vi "LVCAM Propagate Error.vi"(10 "error in":errorcluster, 11 "LVCAM Propagate Error in":refnum<class "LVCAM Propagate Error.lvclass">) -> (0 "error out":errorcluster, 3 "LVCAM Propagate Error out":refnum<class "LVCAM Propagate Error.lvclass">)   [LabVIEW 2021, in "LVCAM.lvlib" / "LVCAM Propagate Error.lvclass"]
uses:
  LVCAM Propagate Error.lvclass
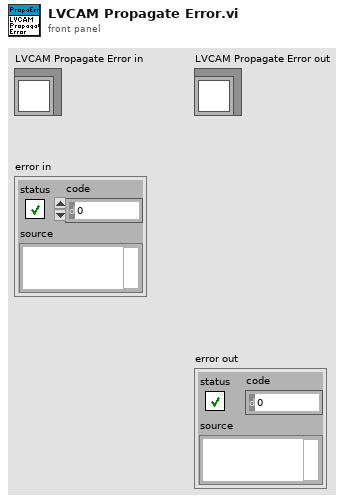
[diagram p1: front panel]
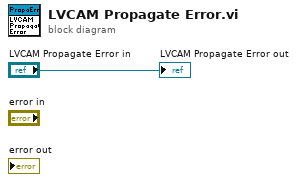
[diagram p0: block diagram]
diagram:
  "LVCAM Propagate Error out" <- "LVCAM Propagate Error in"
